vi "velodyne64.vi"() -> ()   [LabVIEW 2015]
panel:
  in  "Raw LIDAR Data":string
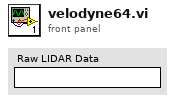
[diagram p1: front panel]
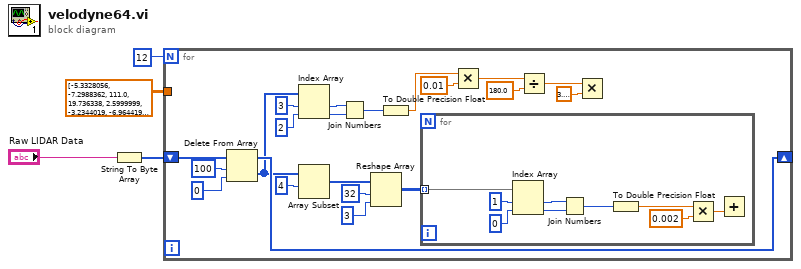
[diagram p0: block diagram]
diagram:
  n1 = String To Byte Array(string="Raw LIDAR Data") -> (unsigned byte array=w3:u8[])
  n2 = for {
    N: 12 -> [_]
    shift-right: [w23] -> _
    shift-left: w3 -> [w26]
    tunnel: dbl[][] [[-5.3328056, -7.2988362, 111.0, 19.736338, 2.5999999], [-3.2344019, -6.9644198, 146.0, 19.778963, -2.5999999], [2.4376695, 0.250889, 131.76823, 20.688799, 2.5999999], [4.7373252, 0.55538797, 138.12656, 20.727015, -2.5999999], [-1.0502493, -6.6410818, 119.0, 19.82012, 2.5999999], [1.2386309, -6.2594609, 135.0, 19.868624, -2.5999999], [-1.8405367, -8.6656351, 132.0, 19.561426, 2.5999999], [0.4511103, -8.3104696, 145.0, 19.606993, -2.5999999], [3.2611551, -5.9352221, 116.0, 19.909781, 2.5999999], [5.4685535, -5.587399, 133.99889, 19.953875, -2.5999999], [2.4743285, -7.9891219, 117.0, 19.648148, 2.5999999], [4.7189918, -7.644258, 145.0, 19.692244, -2.5999999], [-5.3511744, -3.2475569, 118.71672, 20.249313, 2.5999999], [-3.1158857, -2.850472, 142.90839, 20.29929, -2.5999999], [-6.1270261, -5.204318, 120.0, 20.00238, 2.5999999], [-3.852011, -4.9137921, 137.0, 20.039125, -2.5999999], [-1.1109436, -2.4998751, 101.71324, 20.343384, 2.5999999], [1.1519098, -2.184176, 145.31258, 20.38307, -2.5999999], [-1.8682934, -4.5764661, 130.0, 20.081753, 2.5999999], [0.43604341, -4.2038751, 147.0, 20.128786, -2.5999999], [3.1763444, -1.798143, 115.82812, 20.431576, 2.5999999], [5.4284201, -1.49388, 146.0, 20.469791, -2.5999999], [2.4024715, -1.877563, 129.29713, 20.169943, 2.5999999], [4.6698937, -3.492661, 157.97737, 20.218447, -2.5999999], [-5.3977456, 0.88327599, 124.12312, 20.768169, 2.5999999], [-3.1504908, 1.234519, 128.0, 20.812265, -2.5999999], [-6.1759849, -1.177825, 133.0, 20.509478, 2.5999999], [-3.8819003, -0.86169797, 130.0, 20.549164, -2.5999999], [-1.1136208, 1.585669, 131.0, 20.856361, 2.5999999], [1.0969903, 1.925001, 131.0, 20.898987, -2.5999999], [-1.9088749, -0.486963, 138.48773, 20.596197, 2.5999999], [0.36758029, -0.123898, 137.21994, 20.641764, -2.5999999], [-8.3386211, -22.597513, 117.0, 10.828748, 2.5999999], [-4.7629819, -22.397568, 100.0, 10.854152, -2.5999999], [4.1516571, -11.576517, 130.0, 12.142142, 2.5999999], [7.3577185, -10.877901, 102.0, 12.220895, -2.5999999], [-1.2630961, -21.935509, 106.0, 10.912581, 2.5999999], [2.1595552, -21.409546, 91.0, 10.978632, -2.5999999], [-2.6141083, -25.066507, 127.0, 10.508655, 2.5999999], [0.95595688, -24.458101, 95.0, 10.588678, -2.5999999], [5.5369682, -20.777454, 106.0, 11.057385, 2.5999999], [8.9712191, -20.243195, 97.0, 11.123436, -2.5999999], [4.4757471, -23.863358, 115.0, 10.666161, 2.5999999], [7.8848143, -23.352007, 92.0, 10.732212, -2.5999999], [-8.0466499, -16.629311, 135.0, 11.559117, 2.5999999], [-4.595552, -16.230633, 108.0, 11.606115, -2.5999999], [-9.3918352, -19.788239, 135.0, 11.179325, 2.5999999], [-5.9566336, -19.21587, 98.0, 11.249186, -2.5999999], [-1.3779737, -15.754419, 116.0, 11.662004, 2.5999999], [2.0754263, -15.166914, 105.0, 11.730595, -2.5999999], [-2.5654242, -18.828558, 138.0, 11.296184, 2.5999999], [0.87227631, -18.312876, 105.0, 11.358424, -2.5999999], [5.2989287, -14.641928, 123.0, 11.791565, 2.5999999], [8.7970304, -14.048302, 86.0, 11.860156, -2.5999999], [4.1742177, -17.687857, 135.0, 11.433367, 2.5999999], [7.5869775, -17.16544, 92.0, 11.495607, -2.5999999], [-7.8831077, -10.436752, 121.0, 12.270433, 2.5999999], [-4.5919614, -10.085198, 103.0, 12.30981, -2.5999999], [-9.1805763, -13.484814, 146.0, 11.924937, 2.5999999], [-5.7835727, -13.107666, 99.0, 11.968124, -2.5999999], [-1.2335371, -9.5621262, 123.0, 12.368239, 2.5999999], [1.9424959, -9.0374413, 106.0, 12.426669, -2.5999999], [-2.5727935, -12.651329, 134.0, 12.020203, 2.5999999], [0.81118912, -12.115005, 104.0, 12.081173, -2.5999999]] ("Correction Factors") -> [w5]
    n3 = Delete From Array(array=w26, length=100, index=0) -> (deleted portion=w11:u8[], array with subset deleted=w23:u8[])
    n4 = Index Array(array=w11, index #1=3 ("index"), index #2=2 ("index")) -> (element #1=w20:u8, element #2=w19:u8)
    n5 = Array Subset(array=w11, index=4) -> (w9:u8[])  [unwired: 1 in]
    n6 = Join Numbers(hi=w20, lo=w19) -> ((hi.lo)=w18:u16)
    n7 = Reshape Array(w9, 32 ("dimension size"), 3 ("dimension size")) -> (w6:u8[][])
    n8 = To Double Precision Float(number=w18) -> (double precision float=w17:dbl)
    n9 = for {
      tunnel: w6 -> [w35] mode=indexing
      n10 = Index Array(array=w35, index #1=1 ("index"), index #2=0 ("index")) -> (element #1=w31:u8, element #2=w30:u8)
      n11 = Join Numbers(hi=w31, lo=w30) -> ((hi.lo)=w32:u16)
      n12 = To Double Precision Float(number=w32) -> (double precision float=w29:dbl)
      n13 = Multiply(x=w29, y=0.002) -> (x*y=w27:dbl)
      n14 = Add(y=w27) -> ()  [unwired: 1 in, 1 out]
    }
    n15 = Multiply(x=w17, y=0.01) -> (x*y=w15:dbl)
    n16 = Divide(x=w15, y=180.0) -> (x/y=w13:dbl)
    n17 = Multiply(x=w13, y=3.141592653589793) -> ()  [unwired: 1 out]
  }
